vi "Factorial.vi"(1 "n":u16) -> (0 "facgtorial":ext format="%.2f")   [LabVIEW 2018]
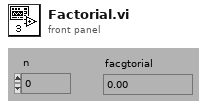
[diagram p1: front panel]
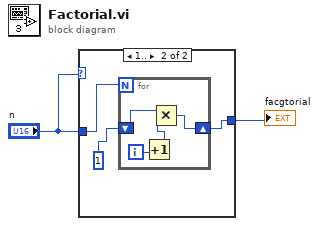
[diagram p0: block diagram]
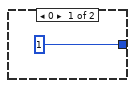
[diagram p2: hidden frame]
diagram:
  n1 = case shown="1.." "n" {
    tunnel: [1 w4] -> w1
    tunnel: "n" -> [_ w6]
    frame 0 {
    }
    frame 1.. {
      n2 = for {
        N: w6 -> [_]
        shift-right: [w7] -> w4
        shift-left: 1 -> [w8]
        i -> [w10]
        n3 = Increment(x=w10) -> (x+1=w9:i32)
        n4 = Multiply(x=w8, y=w9) -> (x*y=w7:i32)
      }
    }
  }
  "facgtorial" <- w1
